vi "Boolean to Unit Vector.vi"(11 "Y Positive":bool) -> (3 "Numeric":i32)   [LabVIEW 2020]
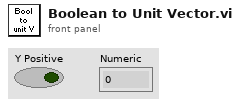
[diagram p1: front panel]
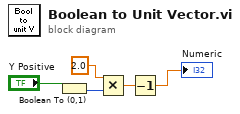
[diagram p0: block diagram]
diagram:
  n1 = Boolean To (0,1)(Boolean="Y Positive") -> (0, 1=w2:i16)
  n2 = Multiply(x=2.0 ("milliseconds to wait"), y=w2) -> (x*y=w1:dbl)
  n3 = Decrement(x=w1) -> (x-1=→"Numeric":dbl)
